vi "TPNT_GetDeviceHelp(all).vi"() -> (2 "help":string)   [LabVIEW 2016]
uses:
  TPNT_DeviceTPs.ctl
  TPNT_TP.ctl
  TPNT_Limits.ctl
  TPNT_Samples.ctl
  TPNT_Log.ctl
panel:
  in  "TPNT_DeviceTPs":T1={"device"="", "devupdate"=0.0, "next_update"=0, "devinterface"="", "TPs"=[], "Alarms"=TRUE, "monitor"=TRUE, "log sep"=""} {"TPs"."Log"."updaterate" format="%.2f"; "TPs"."Samples"."Values" format="%.2f"; "TPs"."Samples"."samples" min=1 step=1; "TPs"."Limits"."Nominal" format="%.2f"; "TPs"."Limits"."Upper" format="%.2f"; "TPs"."Limits"."Lower" format="%.2f"; "TPs"."update_rate" format="%.2f"; "devupdate" format="%.2f"}
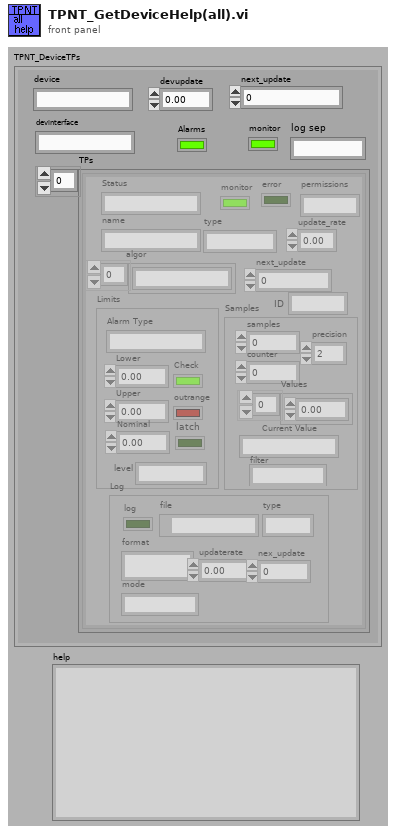
[diagram p1: front panel]
types:
  T1 = typedef "TPNT_DeviceTPs.ctl" = cluster{"device":string, "devupdate":dbl, "next_update":u32, "devinterface":string, "TPs":T2[], "Alarms":bool, "monitor":bool, "log sep":string}
  T2 = typedef "TPNT_TP.ctl" = cluster{"name":string, "type":string, "algor":string[], "update_rate":sgl, "Limits":T3, "Samples":T4, "next_update":u32, "Status":string, "monitor":bool, "error":bool, "Log":T5, "permissions":string, "ID":string}
  T3 = typedef "TPNT_Limits.ctl" = cluster{"Alarm Type":string, "Lower ":dbl, "Upper":dbl, "Nominal":dbl, "outrange":bool, "Check":bool, "latch":bool, "level":string}
  T4 = typedef "TPNT_Samples.ctl" = cluster{"samples":i32, "counter":i32, "Values":dbl[], "Current Value":string, "filter":string, "precision":u8}
  T5 = typedef "TPNT_Log.ctl" = cluster{"log":bool, "file":path, "type":string, "format":string, "updaterate":dbl, "nex_update":u32, "mode":string}
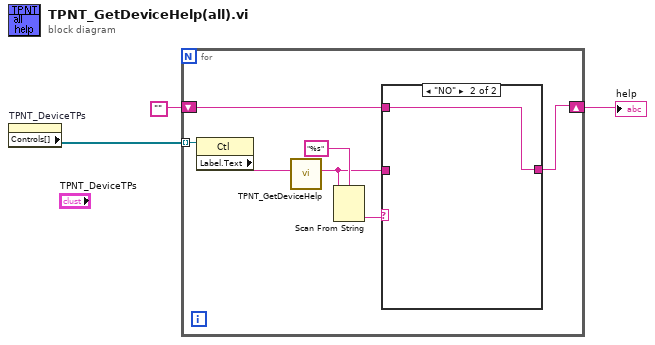
[diagram p0: block diagram]
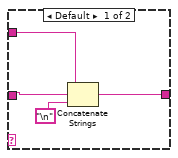
[diagram p2: hidden frame]
diagram:
  n1 = property on="TPNT_DeviceTPs" class="Clust (strict)"() -> ("Controls[]"=w1:refnum<vi>[])  [unwired: 2 in, 2 out]
  n2 = for {
    tunnel: w1 -> [w10] mode=indexing
    shift-right: [w5] -> w2
    shift-left: "" -> [w4]
    n3 = property class="Ctl"(reference=w10) -> ("Label.Text"=w9:string)  [unwired: 1 in, 2 out]
    n4 = call "TPNT_GetDeviceHelp.vi"("name"=w9) -> ("help"=w6:string)  [unwired: 10 out]
    n5 = Scan From String(format string="%s", input string=w6) -> (output 1=w7:string)  [unwired: 2 in, 4 out]
    n6 = case shown="\"NO\"" w7 {
      tunnel: w6 -> [w14 _]
      tunnel: [w12 w15] -> w5
      tunnel: w4 -> [w11 w15]
      frame Default {
        n7 = Concatenate Strings(w11, w14, "\n") -> (w12:string)
      }
      frame "NO" {
      }
    }
  }
  "help" <- w2
